vi "LoadSettingsFromFile.vi"(8 "error in (no error)":errorcluster, 11 "ProgramSettings in":refnum<class "ProgramSettings.lvclass">) -> (0 "error out":errorcluster, 3 "ProgramSettings out":refnum<class "ProgramSettings.lvclass">)   [LabVIEW 2019, in "ProgramSettings.lvclass"]
uses:
  ProgramSettings.lvclass
  ProgramSettings.lvclass/ProgramSettings.ctl
  <vilib>/Utility/xml.llb/Write to XML File(string).vi
  <vilib>/Utility/xml.llb/Read From XML File(string).vi
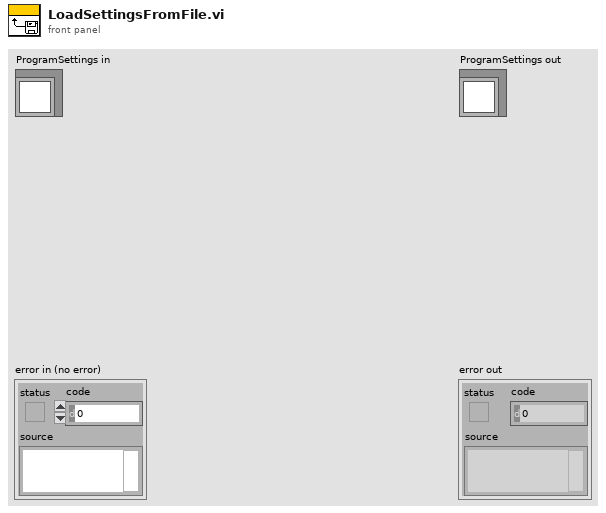
[diagram p1: front panel]
types:
  T1 = typedef "ProgramSettings.lvclass/SettingParams.ctl" = cluster{"Serial Port for strømforsyning":refnum<visa-resource-name>, "Serial Port for SSI Interface":refnum<visa-resource-name>}
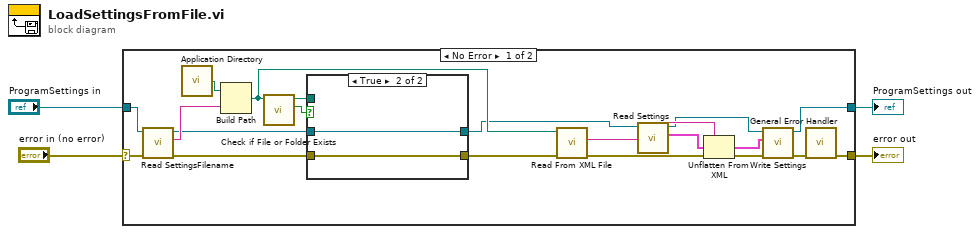
[diagram p0: block diagram]
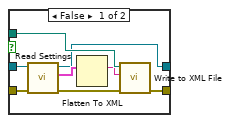
[diagram p2: hidden frame]
diagram:
  n1 = case shown="No Error" "error in (no error)" {
    selector: "error in (no error)" -> [w21 w36]
    tunnel: [w20 w36] -> w3
    tunnel: [w17 w35] -> w1
    tunnel: "ProgramSettings in" -> [w22 w35]
    frame No Error {
      n2 = call "Read SettingsFilename.vi"("error in (no error)"=w21, "ProgramSettings in"=w22) -> ("error out"=w11:errorcluster, "SettingsFilename"=w23:string, "ProgramSettings out"=w12:refnum<class "ProgramSettings.lvclass">)  [unwired: 7 in]
      n3 = call <vilib>:"Application Directory.vi"() -> ("Application Directory"=w16:path)
      n4 = Build Path(base path=w16, name or relative path=w23) -> (appended path=w15:path)
      n5 = call <vilib>:"Check if File or Folder Exists.vi"("path"=w15) -> ("file or folder exists?"=w14:bool, "dup path"=w13:path)  [unwired: 8 in, 1 out]
      n6 = case shown="True" w14 {
        tunnel: w13 -> [w32 _]
        tunnel: w12 -> [w30 w34]
        tunnel: [w29 w34] -> w8
        tunnel: w11 -> [w28 w33]
        tunnel: [w26 w33] -> w10
        frame False {
          n7 = call "Read Settings.vi"("error in (no error)"=w28, "ProgramSettings in"=w30) -> ("error out"=w27:errorcluster, "Settings"=w31:T1, "ProgramSettings out"=w29:refnum<class "ProgramSettings.lvclass">)  [unwired: 7 in]
          n8 = Flatten To XML(anything=w31) -> (xml string=w25:string)
          n9 = call-poly <vilib>:"Write to XML File.vi"("error in (no error)"=w27, "XML Input"=w25, "XML File Path"=w32) -> ("error out"=w26:errorcluster)  [unwired: 6 in, 2 out]
        }
        frame True {
        }
      }
      n10 = call-poly <vilib>:"Read From XML File.vi"("error in (no error)"=w10, "XML File Path"=w15) -> ("error out"=w9:errorcluster, "XML Elements"=w24:string)  [unwired: 7 in, 1 out]
      n11 = call "Read Settings.vi"("ProgramSettings in"=w8) -> ("Settings"=w6:T1, "ProgramSettings out"=w7:refnum<class "ProgramSettings.lvclass">)  [unwired: 8 in, 1 out]
      n12 = Unflatten From XML(xml string=w24, type=w6, error in (no error)=w9) -> (value=w5:T1, error out=w19:errorcluster)
      n13 = call "Write Settings.vi"("error in (no error)"=w19, "Settings"=w5, "ProgramSettings in"=w7) -> ("error out"=w18:errorcluster, "ProgramSettings out"=w17:refnum<class "ProgramSettings.lvclass">)  [unwired: 7 in]
      n14 = call <vilib>:"General Error Handler.vi"("error in (no error)"=w18) -> ("error out"=w20:errorcluster)  [unwired: 10 in, 4 out]
    }
    frame Error {
    }
  }
  "error out" <- w3
  "ProgramSettings out" <- w1
